vi "TDMS Analyse.vi"(8 "Error IN":errorcluster caption="constante d'erreur") -> (0 "Error OUT":errorcluster caption="constante d'erreur")   [LabVIEW 2020]
uses:
  <vilib>/Utility/error.llb/DialogType.ctl
  <vilib>/Utility/TDMS File Viewer/NI_TDMS File Viewer.lvlib
panel:
  out "Error message":string
  in  "Exit Reader":bool
  out "Temperature (°C)":cluster{"Y":dbl[], "Y":dbl[]}[](graph)
  out "YFP (°C)":cluster{"Y":dbl[], "Y":dbl[]}[](graph)
  out "YFP (s)":cluster{"Y":dbl[], "Y":dbl[]}[](graph)
  out "LSSmOrange (°C)":cluster{"Y":dbl[], "Y":dbl[]}[](graph)
  out "LSSmOrange (s)":cluster{"Y":dbl[], "Y":dbl[]}[](graph)
  out "mAmétrine (°C)":cluster{"Y":dbl[], "Y":dbl[]}[](graph)
  out "mAmétrine (s)":cluster{"Y":dbl[], "Y":dbl[]}[](graph)
  out "CFP (°C)":cluster{"Y":dbl[], "Y":dbl[]}[](graph)
  out "CFP (s)":cluster{"Y":dbl[], "Y":dbl[]}[](graph)
  out "Strip lue":string
  out "fichier tdms":refnum<k34>
  out "Nb strip":i32
  out "Lenght":i32
  out "Sample Time (s)":dbl
  in  "Répertoire du fichier TDMS":path=path "D:/Projets/LabView/TiT/test/TDMS/OUT_103123.tdms"
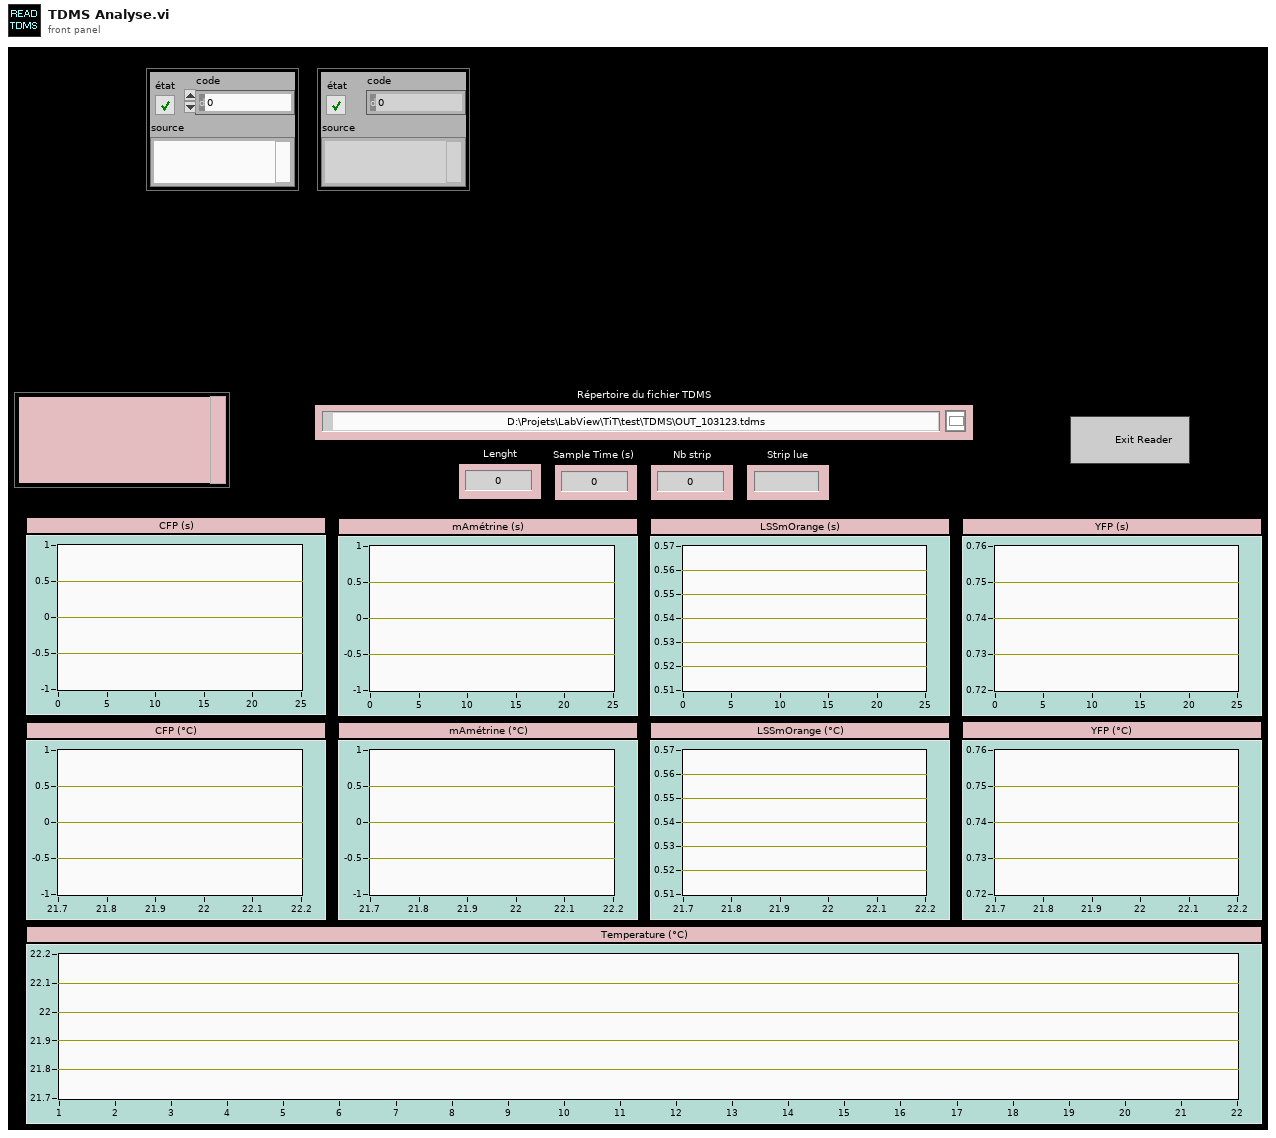
[diagram p1: front panel]
types:
  T1 = enum16{"big-endian, network order", "native, host order", "little-endian"}
  T2 = enum16{"open", "open or create", "create or replace", "create", "open (read-only)"}
  T3 = typedef "DialogType.ctl" = u16
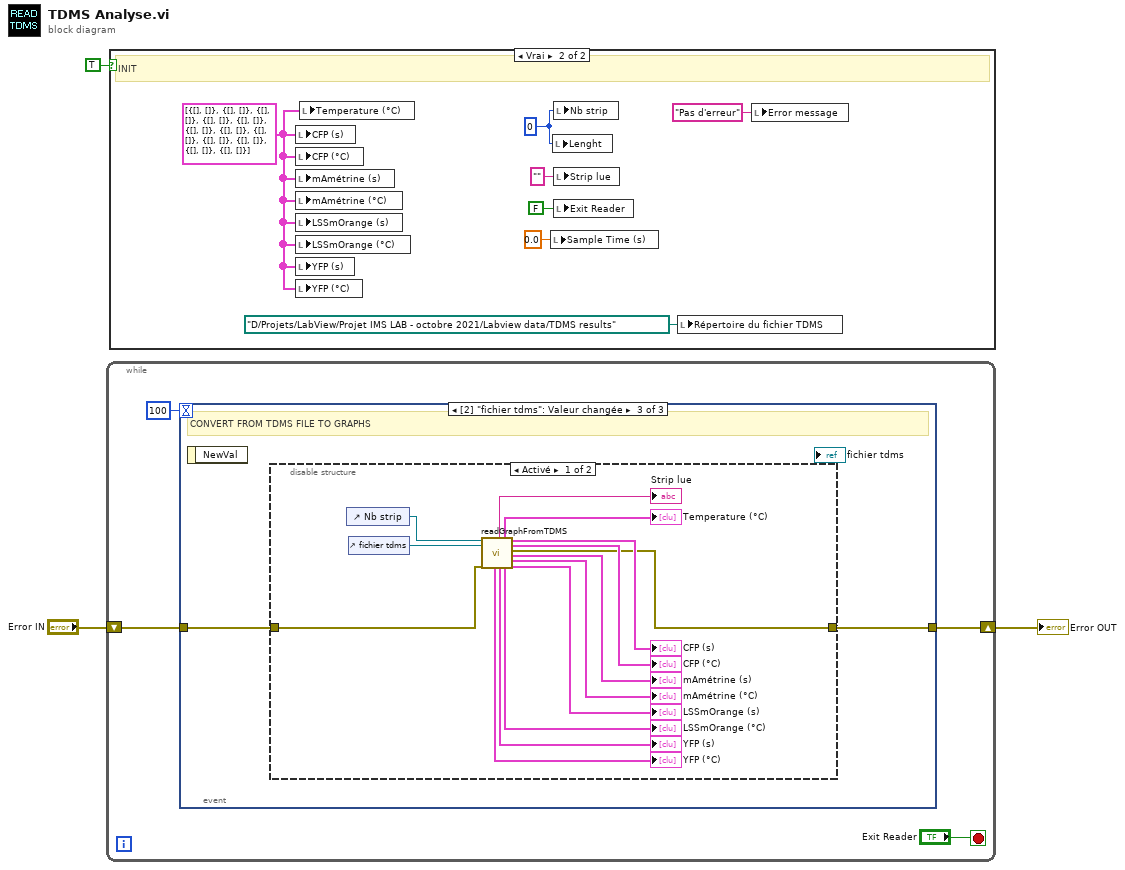
[diagram p0: block diagram]
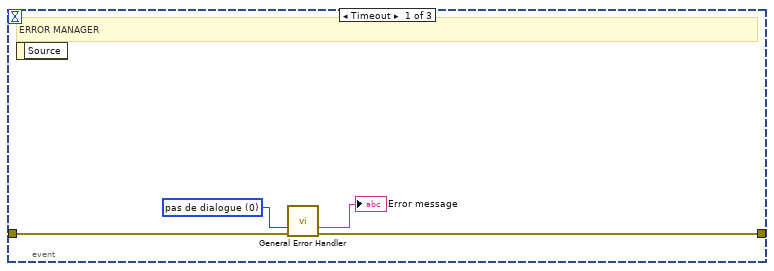
[diagram p3: hidden frame]
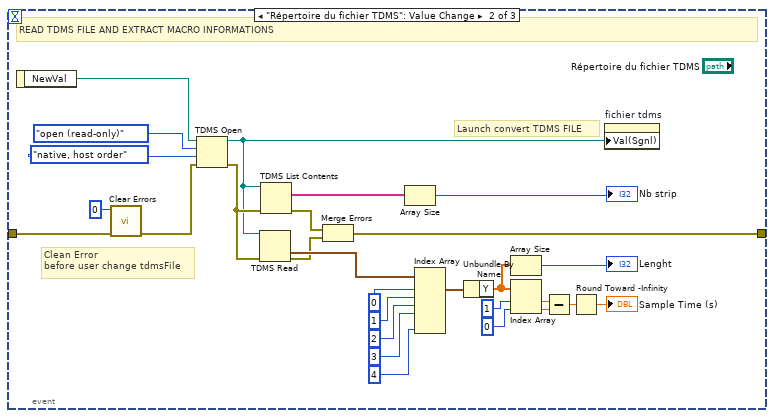
[diagram p4: hidden frame]
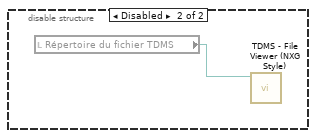
[diagram p5: hidden frame]
diagram:
  n1 = while {
    shift-right: [w4] -> w2
    shift-left: "Error IN" -> [w6]
    stop <- "Exit Reader" stop-if-true
    n2 = event shown="[2] \"fichier tdms\": Valeur changée" {
      selector: _ -> [_ _ _]
      dyn-events: _ -> [_ _ _]
      timeout: 100 -> [_ _ _]
      tunnel: w6 -> [w11 w15 w41]
      tunnel: [w8 w12 w40] -> w4
      event Timeout {
        w10 = T3 0 items=["pas de dialogue", "Message OK", "Message continuer ou arrêter", "Message OK + mises en garde", "Arrêter/Continuer + mises en garde"] ("type of dialog (OK msg:1)")
        # "ERROR MANAGER"
        n3 = event-data() -> ()  [unwired: 1 in, 1 out]
        n4 = call <vilib>:"General Error Handler.vi"("type of dialog (OK msg:1)"=w10, "error in (no error)"=w11) -> ("message"=→"Error message":string, "error out"=w8:errorcluster)  [unwired: 9 in, 3 out]
      }
      event "Répertoire du fichier TDMS": Value Change {
        # "Launch convert TDMS FILE"
        # "Clean Error\nbefore user change tdmsFile"
        # "READ TDMS FILE AND EXTRACT MACRO INFORMATIONS"
        n5 = event-data() -> ("NewVal"=w37:path)  [unwired: 1 in]
        n6 = call <vilib>:"Clear Errors.vi"("error in (no error)"=w15, "specific error code to clear (0: all)"=0) -> ("error out"=w14:errorcluster)  [unwired: 4 in, 1 out]
        n7 = TDMS Open(8:w14, 9:T1."native, host order" ("ordre des octets (2 : Little Endian)"), 10:T2."open (read-only)" ("opération (0 : open)"), 11:w37) -> (0:w19:errorcluster, 3:w16:refnum<k34>)  [unwired: 3 in]
        n8 = TDMS Read(0:w16, 11:w19) -> (10:w20:waveform(dbl)[], 15:w17:errorcluster)  [unwired: 6 in, 4 out]
        n9 = TDMS List Contents(4:w19, 7:w16) -> (0:w18:errorcluster, 2:w35:string[])  [unwired: 1 in, 2 out]
        n10 = Merge Errors(w18, w17) -> (w12:errorcluster)
        n11 = Array Size(array=w35) -> (size(s)=→"Nb strip":i32)
        n12 = Index Array(array=w20, index #1=0 ("indice"), index #2=1 ("indice"), index #3=2 ("indice"), index #4=3 ("indice"), index #6=4 ("indice")) -> (element #1=w26:waveform(dbl))  [unwired: 1 in, 5 out]
        n13 = Unbundle By Name(w26) -> ("Y"=w33:dbl[])
        n14 = Array Size(array=w33) -> (size(s)=→"Lenght":i32)
        n15 = Index Array(array=w33, index #1=1 ("indice"), index #2=0 ("indice")) -> (element #1=w30:dbl, element #2=w29:dbl)
        n16 = Subtract(x=w30, y=w29) -> (x-y=w31:dbl)
        n17 = Round Toward -Infinity(1:w31) -> (0:→"Sample Time (s)":dbl)
        n18 = property on="fichier tdms" class="Ref (strict)"("Val(Sgnl)"=w16) -> ()  [unwired: 2 in, 2 out]
      }
      event "fichier tdms": Value Change {
        # "CONVERT FROM TDMS FILE TO GRAPHS"
        n19 = event-data() -> ()  [unwired: 1 in, 1 out]
        n20 = disable-structure shown="Activé" {
          disable-tunnel: w41 -> [w43 _]
          disable-tunnel: [w42 _] -> w40
          frame Enabled {
            n21 = control-ref of="Nb strip"() -> (w55:refnum<vi>)
            n22 = control-ref of="fichier tdms"() -> (w54:refnum<vi>)
            n23 = call "readGraphFromTDMS.vi"("Refnum NumNb"=w55, "Refnum en entrée"=w54, "Error IN"=w43) -> ("YFP (°C)"=→"YFP (°C)":cluster{"Y":dbl[], "Y":dbl[]}[], "Strip lue"=→"Strip lue":string, "YFP (s)"=→"YFP (s)":cluster{"Y":dbl[], "Y":dbl[]}[], "TEMPERATURE (°C)"=→"Temperature (°C)":cluster{"Y":dbl[], "Y":dbl[]}[], "LSSmOrange (°C)"=→"LSSmOrange (°C)":cluster{"Y":dbl[], "Y":dbl[]}[], "CFP (s)"=→"CFP (s)":cluster{"Y":dbl[], "Y":dbl[]}[], "CFP (°C)"=→"CFP (°C)":cluster{"Y":dbl[], "Y":dbl[]}[], "Error OUT"=w42:errorcluster, "mAmétrine (s)"=→"mAmétrine (s)":cluster{"Y":dbl[], "Y":dbl[]}[], "mAmétrine (°C)"=→"mAmétrine (°C)":cluster{"Y":dbl[], "Y":dbl[]}[], "LSSmOrange (s)"=→"LSSmOrange (s)":cluster{"Y":dbl[], "Y":dbl[]}[])  [unwired: 6 in]
          }
          frame Disabled {
            n24 = local read "Répertoire du fichier TDMS"() -> (w56:path)
            n25 = call <vilib>:"TDMS - File Viewer (NXG Style).vi"("file in"=w56) -> ()  [unwired: 9 in, 2 out]
          }
        }
      }
    }
  }
  "Error OUT" <- w2
  n26 = case shown="Vrai" TRUE {
    frame False {
    }
    frame True {
      w59 = 0 ("Lenght")
      w62 = cluster{"Y":dbl[], "Y":dbl[]}[] [{"Y"=[], "Y"=[]}, {"Y"=[], "Y"=[]}, {"Y"=[], "Y"=[]}, {"Y"=[], "Y"=[]}, {"Y"=[], "Y"=[]}, {"Y"=[], "Y"=[]}, {"Y"=[], "Y"=[]}, {"Y"=[], "Y"=[]}, {"Y"=[], "Y"=[]}, {"Y"=[], "Y"=[]}, {"Y"=[], "Y"=[]}, {"Y"=[], "Y"=[]}] ("CFP (s)")
      # "INIT"
      n27 = local write "CFP (s)"(w62) -> ()
      n28 = local write "CFP (°C)"(w62) -> ()
      n29 = local write "mAmétrine (s)"(w62) -> ()
      n30 = local write "mAmétrine (°C)"(w62) -> ()
      n31 = local write "LSSmOrange (s)"(w62) -> ()
      n32 = local write "LSSmOrange (°C)"(w62) -> ()
      n33 = local write "YFP (s)"(w62) -> ()
      n34 = local write "YFP (°C)"(w62) -> ()
      n35 = local write "Temperature (°C)"(w62) -> ()
      n36 = local write "Sample Time (s)"(0.0 ("Sample Time (s)")) -> ()
      n37 = local write "Lenght"(w59) -> ()
      n38 = local write "Nb strip"(w59) -> ()
      n39 = local write "Strip lue"("" ("Strip lue")) -> ()
      n40 = local write "Exit Reader"(FALSE ("Exit Reader")) -> ()
      n41 = local write "Répertoire du fichier TDMS"(path "D:/Projets/LabView/Projet IMS LAB - octobre 2021/Labview data/TDMS results" ("Répertoire du fichier TDMS")) -> ()
      n42 = local write "Error message"("Pas d'erreur" ("Error message")) -> ()
    }
  }
